vi "Main.vi"(8 "error in":errorcluster, 11 "Container in":refnum<class "Container.lvclass">) -> (0 "error out":errorcluster, 3 "Container out":refnum<class "Container.lvclass">)   [LabVIEW 2023, in "Container.lvclass"]
doc: "The Queued Message Handler of a Worker."
uses:
  Container.lvclass
  C:/Program Files (x86)/National Instruments/LabVIEW 2023/vi.lib/addons/_Workers/Library/Classes/Worker/Worker.lvclass
  System.Windows.Forms
  Container.lvclass/Container.ctl
  <vilib>/addons/_Workers/Library/Classes/Worker/Worker.lvclass/Worker.ctl
  Worker-1/Worker-1.lvclass
  <userlib>/LV-TOML/lib/Write TOML File (TOML).vi
  <vilib>/addons/_Workers/Library/Classes/Message/Enqueue Message to Queue.vi
  <vilib>/addons/_Workers/Library/Classes/Message/Enqueue Message to Self v2.vi
  <vilib>/MGI/Panel Manager - .NET Panels/MDI/MDI Container/MDI Container.lvclass
  <vilib>/MGI/Panel Manager/Panel/Panel/Window/Window.lvclass
  UI Cam Basler/UI Cam Basler.lvclass
  Initialization Data.ctl
  <vilib>/addons/_Workers/Library/Classes/Worker/Worker.lvclass
  <vilib>/addons/_Workers/Debugger/Debug Client/Debug Client.lvlib
  <vilib>/addons/_Workers/Library/Classes/Message/Message.lvclass
  <userlib>/LV-TOML/lib/LV-TOML.lvlib
  C:/Program Files (x86)/National Instruments/LabVIEW 2023/vi.lib/addons/_Workers/Library/Classes/Workers Object/Workers Object.lvclass
  C:/Users/flepetit/Desktop/CamView-mdi-LV/Workers/Container/Container.lvclass
  C:/Users/flepetit/Desktop/CamView-mdi-LV/Workers/Worker-1/Worker-1.lvclass
panel:
  in  "Camera monitoring container":refnum<k24>(container)
  out "Caméra CL":bool
  in  "Plac.Hor.":bool
  in  "Plac.Vert.":bool
  out "Caméra CP":bool
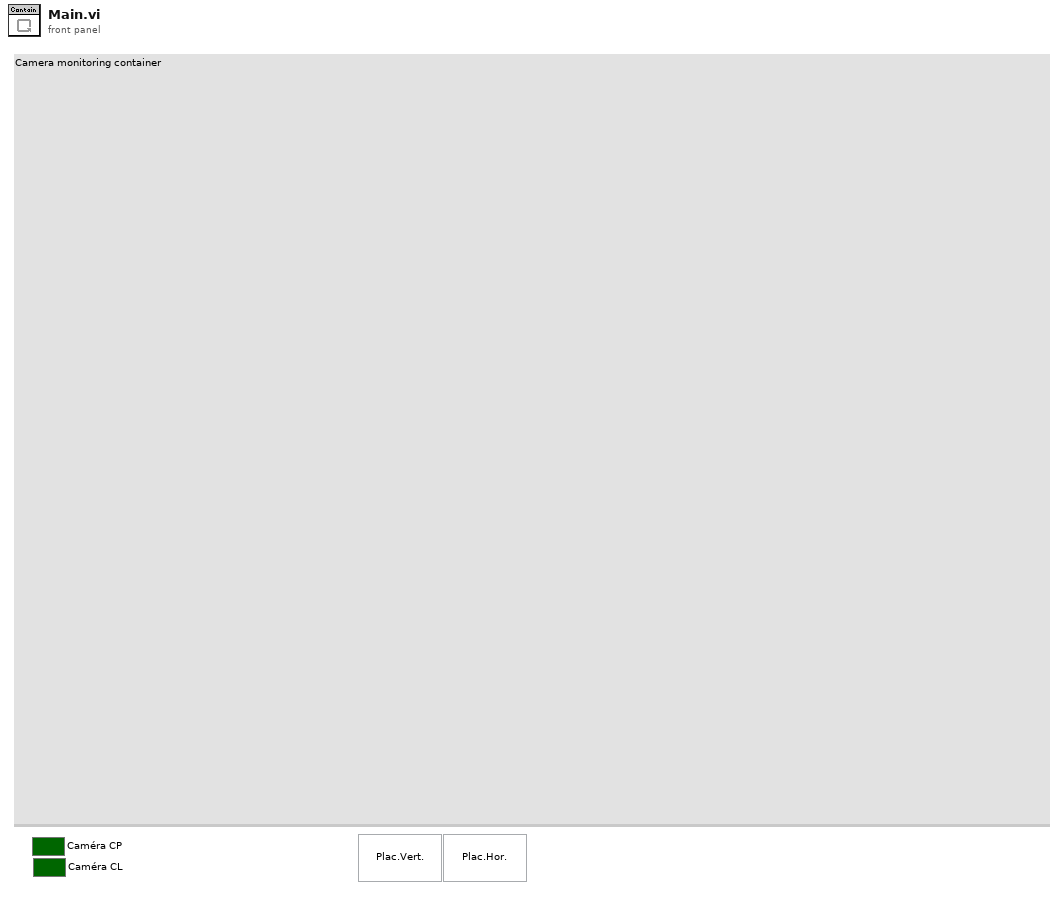
[diagram p1: front panel]
types:
  T1 = typedef "Container.lvclass/Initialization Data.ctl" = cluster{"String":string}
  T2 = typedef "Container.lvclass/Parsed data container.ctl" = cluster{"Ctrl Config":cluster{"Caméra CP":bool, "Caméra CL":bool}}
  T3 = typedef "LV-TOML.lvlib/TOML Value.ctl" = cluster{"type":enum16{"Table", "Array", "String", "Integer", "Float", "Boolean", "Offset Date-Time", "Local Date-Time", "Local Date", "Local Time", "Path"}, "value":variant}
  T4 = typedef "Workers.lvlib/Case Label.ctl" = string
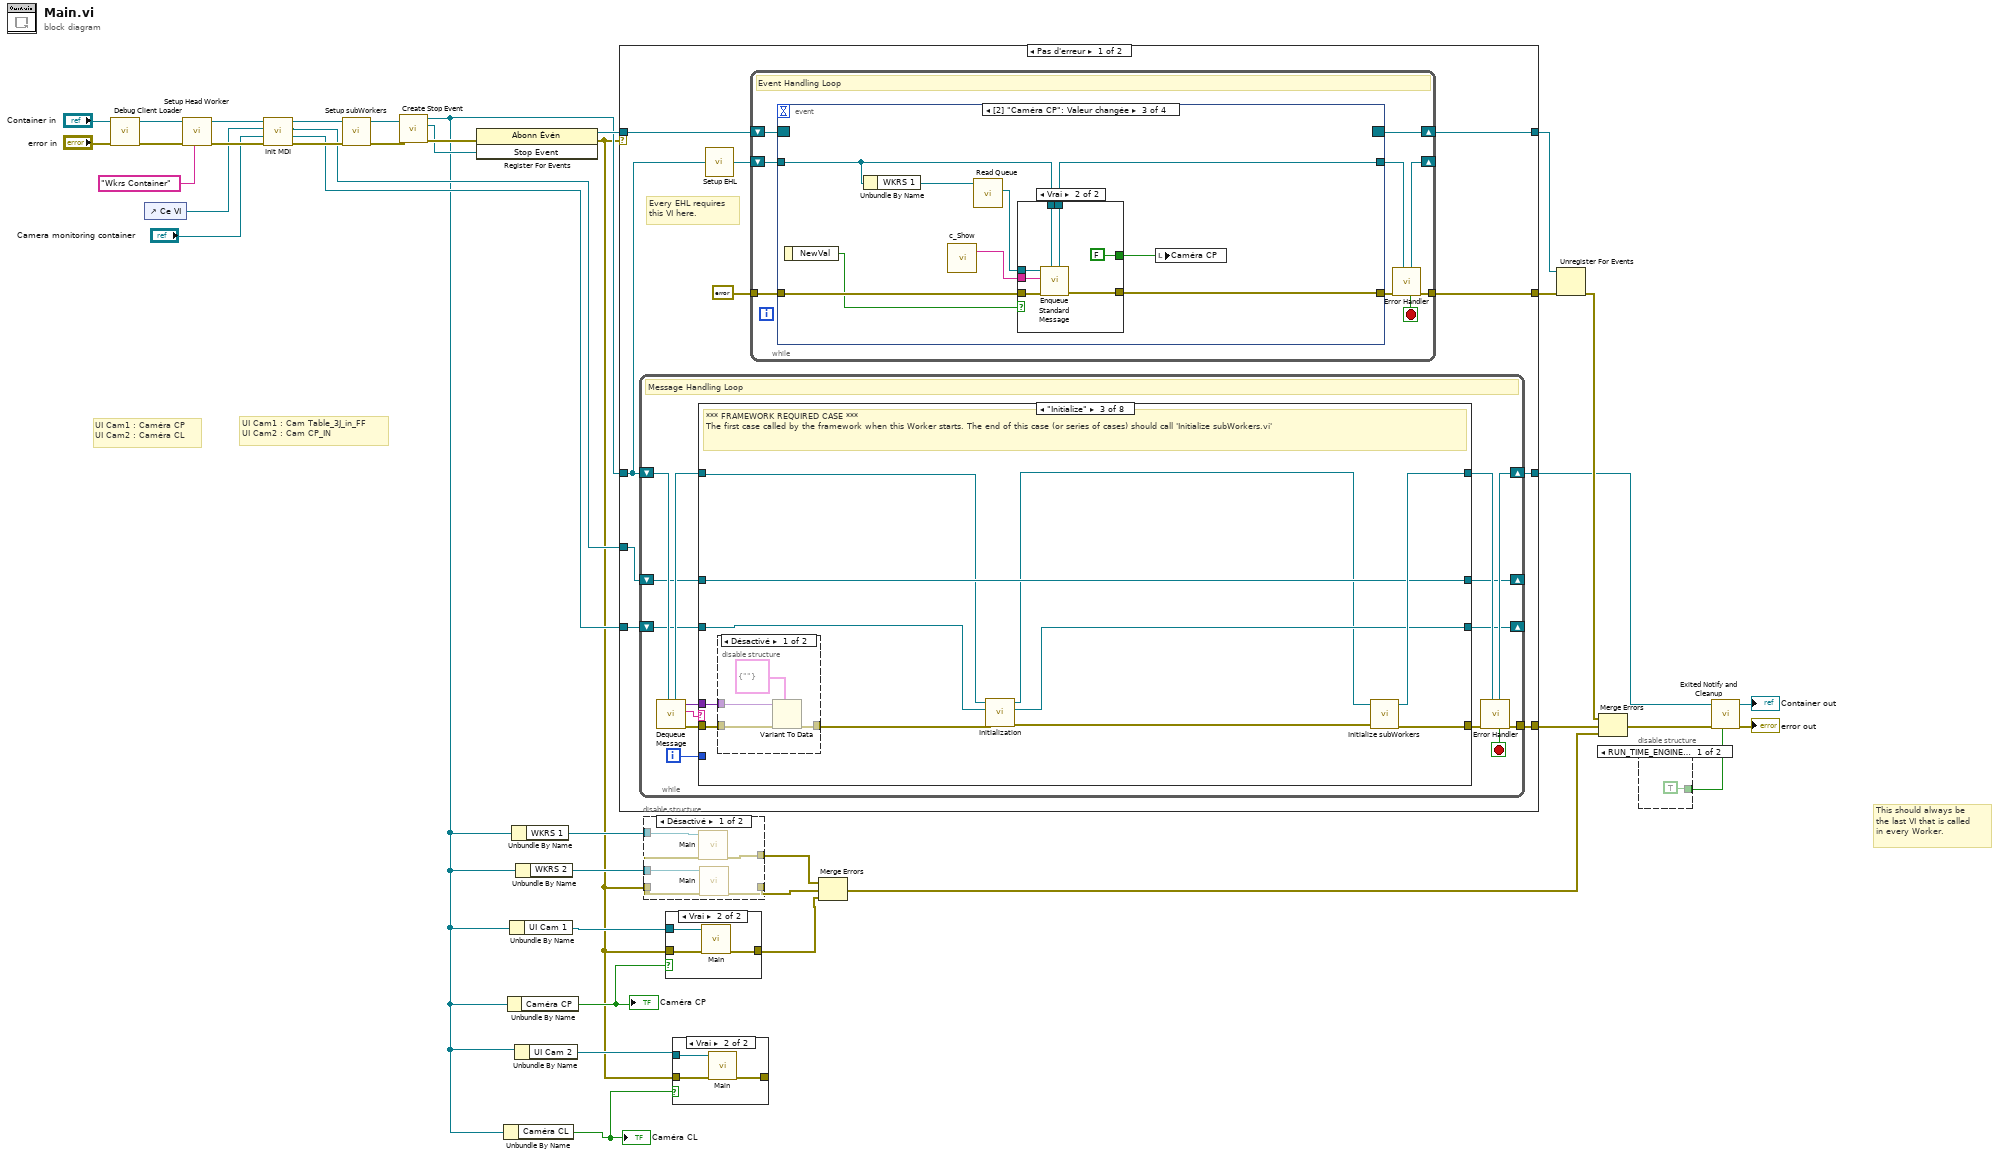
[diagram p0: block diagram]
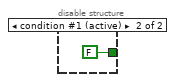
[diagram p2: hidden frame]
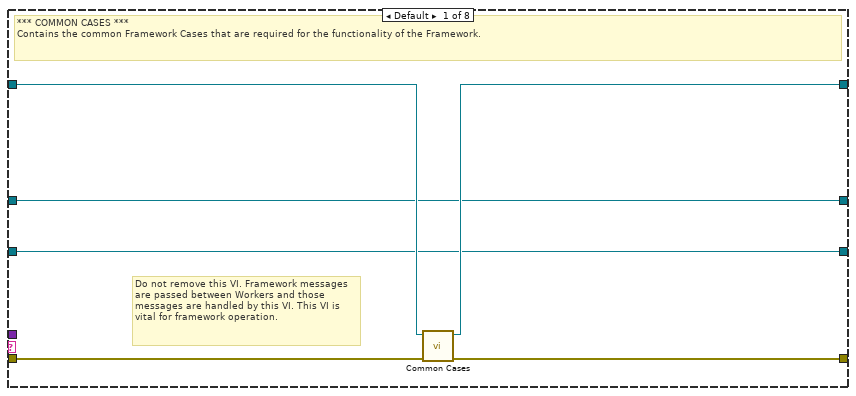
[diagram p6: hidden frame]
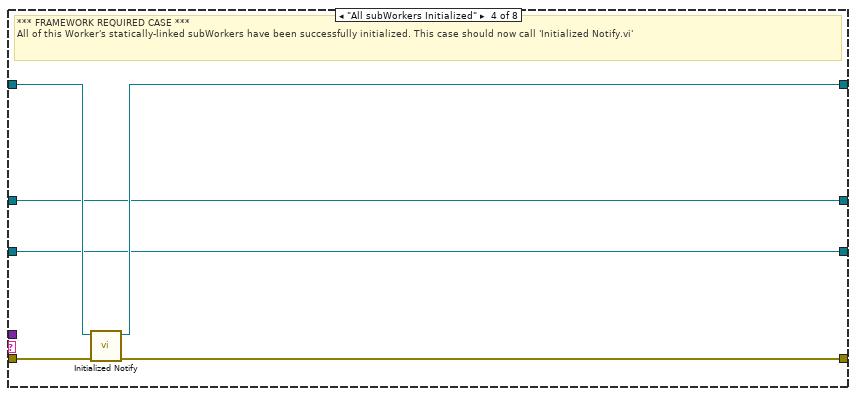
[diagram p9: hidden frame]
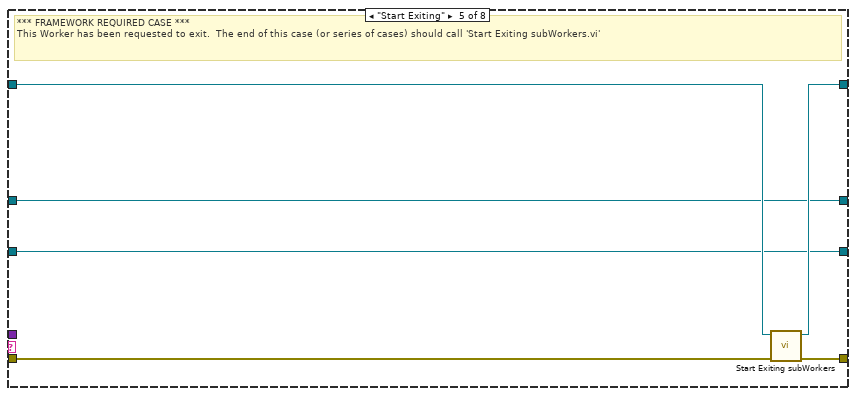
[diagram p10: hidden frame]
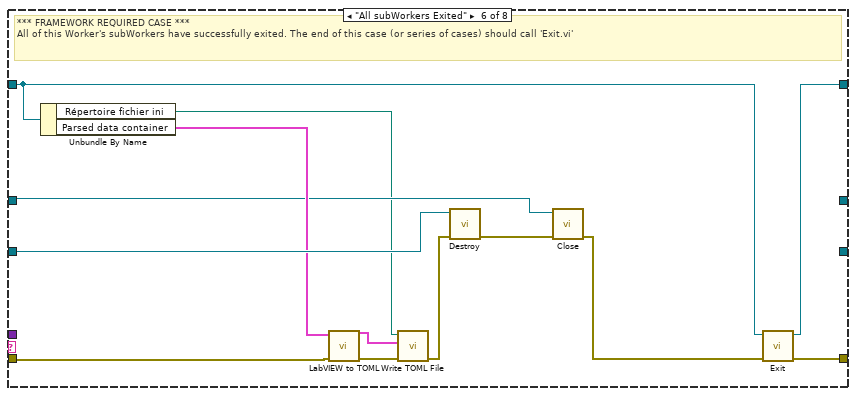
[diagram p11: hidden frame]
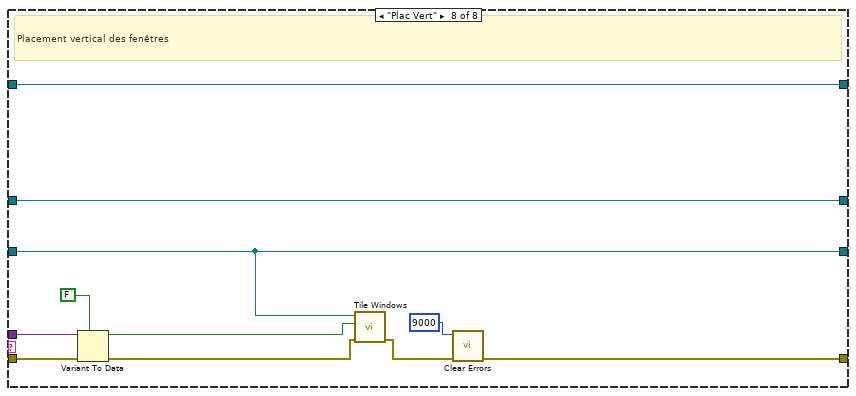
[diagram p13: hidden frame]
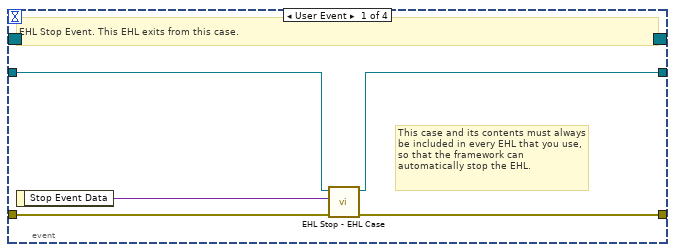
[diagram p14: hidden frame]
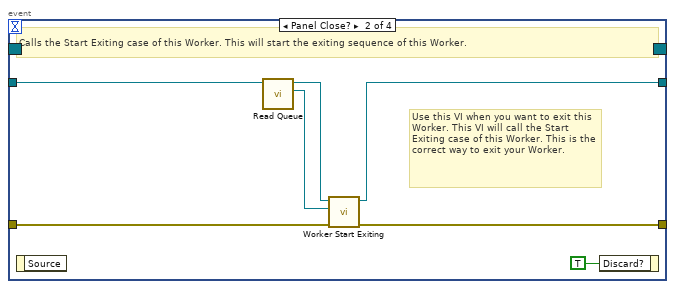
[diagram p15: hidden frame]
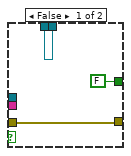
[diagram p16: hidden frame]
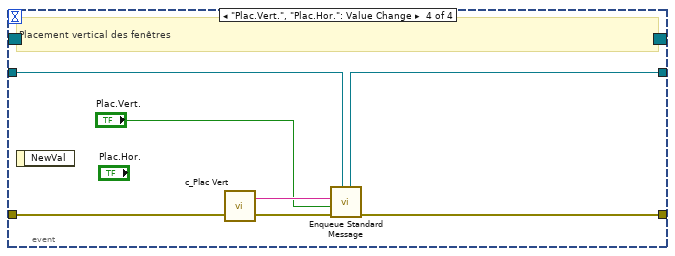
[diagram p17: hidden frame]
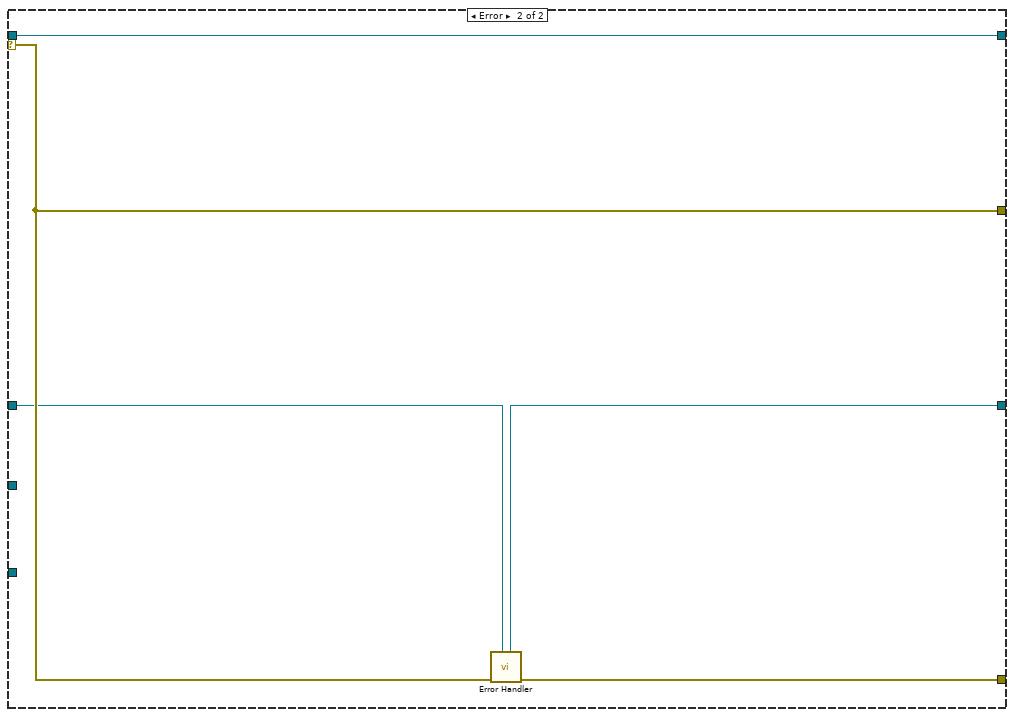
[diagram p18: hidden frame]
diagram:
  # "UI Cam1 : Cam Table_3J_in_FF\nUI Cam2 : Cam CP_IN"
  # "UI Cam1 : Caméra CP\nUI Cam2 : Caméra CL"
  # "This should always be the last VI that is called in every Worker."
  n1 = call <vilib>:"Debug Client Loader.vi"("error in (no error)"="error in", "Worker"="Container in") -> ("error out"=w24:errorcluster, "Worker out"=w23:refnum<class "Container.lvclass">)  [unwired: 8 in]
  n2 = control-ref of="Ce VI"() -> (w9:refnum<vi>)
  n3 = call-dynamic "Setup Head Worker.vi"("Worker Alias"="Wkrs Container", "error in"=w24, "Worker"=w23) -> ("error out"=w15:errorcluster, "Worker out"=w12:refnum<class "Container.lvclass">)  [unwired: 7 in]
  n4 = call "Init MDI.vi"("error in (no error)"=w15, "Camera monitoring container"="Camera monitoring container", "Refnum VI"=w9, "Container en entrée"=w12) -> ("error out"=w14:errorcluster, "Container out"=w10:refnum<class "MDI Container.lvclass">, "Panel Out"=w11:refnum<class "Window.lvclass">, "Container en sortie"=w13:refnum<class "Container.lvclass">)  [unwired: 4 in]
  n5 = call "Setup subWorkers.vi"("error in"=w14, "Container in"=w13) -> ("error out"=w21:errorcluster, "Container out"=w22:refnum<class "Container.lvclass">)  [unwired: 8 in]
  n6 = call-dynamic "Create Stop Event.vi"("error in"=w21, "Worker"=w22) -> ("error out"=w34:errorcluster, "Stop Event"=w31:refnum<user-event>, "Worker out"=w6:refnum<class "Container.lvclass">)  [unwired: 7 in]
  n7 = register-events(error in=w34, w31) -> (reference out=w33:refnum<event-registration>, error out=w4:errorcluster)  [unwired: 1 in]
  n8 = Unbundle By Name(w6) -> ("Caméra CL"=w3:bool)
  "Caméra CL" <- w3
  n9 = Unbundle By Name(w6) -> ("Caméra CP"=w7:bool)
  "Caméra CP" <- w7
  n10 = Unbundle By Name(w6) -> ("UI Cam 1"=w17:refnum<class "UI Cam Basler.lvclass">)
  n11 = Unbundle By Name(w6) -> ("WKRS 1"=w27:refnum<class "Worker-1.lvclass">)
  n12 = Unbundle By Name(w6) -> ("UI Cam 2"=w5:refnum<class "UI Cam Basler.lvclass">)
  n13 = Unbundle By Name(w6) -> ("WKRS 2"=w19:refnum<class "Worker-1.lvclass">)
  n14 = case shown="Pas d'erreur" w4 {
    tunnel: w6 -> [w44 w178]
    tunnel: [w42 w179] -> w32
    tunnel: w33 -> [w49 w180]
    tunnel: [w46 w181] -> w38
    tunnel: [w48 w180] -> w37
    tunnel: [w43 w177] -> w35
    selector: w4 -> [_ w181]
    tunnel: w11 -> [w41 _]
    tunnel: w10 -> [w40 _]
    frame No Error {
      # "Every EHL requires\nthis VI here."
      n15 = while {
        shift-right: [w62] -> w43
        shift-left: w44 -> [w64]
        tunnel: [w63] -> w42
        shift-right: [w53] -> _
        shift-left: w41 -> [w52]
        shift-right: [w51] -> _
        shift-left: w40 -> [w50]
        i -> [w54]
        stop <- w55 stop-if-true
        # "Message Handling Loop"
        n16 = call-dynamic "Dequeue Message.vi"("Worker"=w64) -> ("error out"=w61:errorcluster, "Case out"=w56:string, "Data out"=w57:variant, "Worker out"=w59:refnum<class "Container.lvclass">)  [unwired: 6 in, 1 out]
        n17 = case "Worker MHL Case Structure (DO NOT CHANGE LABEL NAME)" shown="\"Initialize\"" w56 {
          tunnel: w61 -> [w70 w73 w83 w94 w99 w108 w118 w128]
          tunnel: [w69 w73 w85 w93 w102 w115 w118 w121] -> w60
          tunnel: w59 -> [w68 w74 w76 w96 w100 w104 w119 w130]
          tunnel: [w67 w74 w84 w95 w101 w114 w119 w130] -> w58
          tunnel: w57 -> [_ _ w82 _ _ _ _ w127]
          tunnel: w54 -> [_ _ _ _ _ _ _ _]
          tunnel: [w66 w72 w81 w92 w98 _ w117 w129] -> w53
          tunnel: w52 -> [w66 w72 w81 w92 w98 w105 w117 w129]
          tunnel: [w65 w71 w77 w91 w97 _ w116 w120] -> w51
          tunnel: w50 -> [w65 w71 w78 w91 w97 w111 w116 w120]
          frame Default {
            # "Do not remove this VI. Framework messages are passed between Workers and those messages are handled by this VI. This VI is vital for framework operation."
            # "*** COMMON CASES ***\nContains the common Framework Cases that are required for the functionality of the Framework."
            n18 = call-dynamic "Common Cases.vi"("error in"=w70, "Worker in"=w68) -> ("error out"=w69:errorcluster, "Worker out"=w67:refnum<class "Container.lvclass">)  [unwired: 8 in]
          }
          frame "------ FRAMEWORK REQUIRED CASES ------" {
            # "Start of Framework Required Cases"
          }
          frame "Initialize" {
            # "*** FRAMEWORK REQUIRED CASE ***\nThe first case called by the framework when this Worker starts. The end of this case (or series of cases) should call 'Initialize subWorkers.vi'"
            n19 = disable-structure shown="Désactivé" {
              disable-tunnel: w83 -> [w89 w90]
              disable-tunnel: [w88 w90] -> w80
              disable-tunnel: w82 -> [w87 _]
              frame Disabled {
                n20 = Variant To Data(error in=w89, type=T1 {"String"=""} ("Initialization Data"), Variant=w87) -> (error out=w88:errorcluster)  [unwired: 1 out]
              }
              frame Enabled {
              }
            }
            n21 = call "Initialization.vi"("error in (no error)"=w80, "Container in"=w78, "Container en entrée"=w76) -> ("error out"=w79:errorcluster, "Container out"=w77:refnum<class "MDI Container.lvclass">, "Container en sortie"=w75:refnum<class "Container.lvclass">)  [unwired: 6 in]
            n22 = call-dynamic "Initialize subWorkers.vi"("error in"=w79, "Worker"=w75) -> ("error out"=w85:errorcluster, "dup Worker out"=w84:refnum<class "Container.lvclass">)  [unwired: 8 in]
          }
          frame "All subWorkers Initialized" {
            # "*** FRAMEWORK REQUIRED CASE ***\nAll of this Worker's statically-linked subWorkers have been successfully initialized. This case should now call 'Initialized Notify.vi'"
            n23 = call-dynamic "Initialized Notify.vi"("error in"=w94, "Worker"=w96) -> ("error out"=w93:errorcluster, "dup Worker out"=w95:refnum<class "Container.lvclass">)  [unwired: 8 in]
          }
          frame "Start Exiting" {
            # "*** FRAMEWORK REQUIRED CASE ***\nThis Worker has been requested to exit.  The end of this case (or series of cases) should call 'Start Exiting subWorkers.vi'"
            n24 = call-dynamic "Start Exiting subWorkers.vi"("error_in"=w99, "Worker"=w100) -> ("error out"=w102:errorcluster, "dup Worker out"=w101:refnum<class "Container.lvclass">)  [unwired: 8 in]
          }
          frame "All subWorkers Exited" {
            # "*** FRAMEWORK REQUIRED CASE ***\nAll of this Worker's subWorkers have successfully exited. The end of this case (or series of cases) should call 'Exit.vi'"
            n25 = Unbundle By Name(w104) -> ("Répertoire fichier ini"=w103:path, "Parsed data container"=w106:T2)
            n26 = call <userlib>:"LabVIEW to TOML.vi"("error in (no error)"=w108, "LV Value"=w106) -> ("error out"=w109:errorcluster, "TOML Value"=w110:T3)  [unwired: 7 in, 1 out]
            n27 = call-poly <userlib>:"Write TOML File.vi"("error in (no error)"=w109, "Value"=w110, "file path (use dialog)"=w103) -> ("error out"=w107:errorcluster)  [unwired: 8 in]
            n28 = call <vilib>:"Destroy.vi"("error in (no error)"=w107, "Container in"=w111) -> ("error out"=w113:errorcluster)  [unwired: 9 in]
            n29 = call-dynamic "Close.vi"("error in (no error)"=w113, "UI Element in"=w105) -> ("error out"=w112:errorcluster)  [unwired: 9 in]
            n30 = call-dynamic "Exit.vi"("error_in"=w112, "Worker"=w104) -> ("error out"=w115:errorcluster, "dup Worker out"=w114:refnum<class "Container.lvclass">)  [unwired: 8 in]
          }
          frame "------------------Himself---------------------------" {
            # "End of Framework Required Cases"
          }
          frame "Plac Vert" {
            # "Placement vertical des fenêtres"
            n31 = Variant To Data(error in=w128, type=FALSE, Variant=w127) -> (data=w125:bool, error out=w124:errorcluster)
            n32 = call <vilib>:"Tile Windows.vi"("error in (no error)"=w124, "Vertical?"=w125, "Container in"=w120) -> ("error out"=w122:errorcluster)  [unwired: 8 in]
            n33 = call <vilib>:"Clear Errors.vi"("error in (no error)"=w122, "specific error code to clear (0: all)"=9000) -> ("error out"=w121:errorcluster)  [unwired: 4 in, 1 out]
          }
        }
        n34 = call-dynamic "Error Handler.vi"("Worker"=w58, "error_in"=w60) -> ("error out"=w63:errorcluster, "Stop Loop"=w55:bool, "Worker out"=w62:refnum<class "Container.lvclass">)  [unwired: 7 in]
      }
      n35 = call-dynamic "Setup EHL.vi"("Worker"=w44) -> ("Worker out"=w45:refnum<class "Container.lvclass">)  [unwired: 14 in]
      n36 = while "Event Handling Loop" {
        shift-right: [w139] -> w48
        shift-left: w49 -> [w138]
        tunnel: [w134] -> w46
        tunnel: errorcluster {"status"=FALSE, "code"=0, "source"=""} ("error constant") -> [w136]
        shift-right: [w132] -> _
        shift-left: w45 -> [w137]
        stop <- w131 stop-if-true
        # "Event Handling Loop"
        n37 = event shown="[2] \"Caméra CP\": Valeur changée" {
          selector: w138 -> [_ _ _ _]
          dyn-events: [_ _ _ _] -> w139
          timeout: _ -> [_ _ _ _]
          tunnel: [w143 w150 w158 w173] -> w135
          tunnel: w136 -> [w144 w149 w160 w174]
          tunnel: w137 -> [w142 w148 w157 w176]
          tunnel: [w141 w147 w159 w175] -> w133
          event User Event {
            # "This case and its contents must always be included in every EHL that you use, so that the framework can automatically stop the EHL."
            # "EHL Stop Event. This EHL exits from this case."
            n38 = event-data() -> ("Stop Event Data"=w140:variant)  [unwired: 1 in]
            n39 = call <vilib>:"EHL Stop - EHL Case.vi"("error in"=w144, "Stop Event Data"=w140, "Worker"=w142) -> ("error out"=w143:errorcluster, "Worker out"=w141:refnum<class "Container.lvclass">)  [unwired: 7 in]
          }
          event Panel Close? {
            # "Use this VI when you want to exit this Worker. This VI will call the Start Exiting case of this Worker. This is the correct way to exit your Worker."
            # "Calls the Start Exiting case of this Worker. This will start the exiting sequence of this Worker."
            n40 = event-data() -> ()  [unwired: 1 in, 1 out]
            n41 = call <vilib>:"Read Queue.vi"("Worker"=w148) -> ("Message Queue out"=w145:refnum<class "Message Queue.lvclass">, "dup Worker out"=w146:refnum<class "Container.lvclass">)  [unwired: 9 in]
            n42 = call-dynamic "Worker Start Exiting.vi"("error_in"=w149, "Message Queue"=w145, "Worker"=w146) -> ("error out"=w150:errorcluster, "dup Worker out"=w147:refnum<class "Container.lvclass">)  [unwired: 7 in]
            n43 = event-data ("Nœud de filtre d'événements")("Discard?"=TRUE) -> ()  [unwired: 1 in, 1 out]
          }
          event "Caméra CP": Value Change {
            n44 = event-data() -> ("NewVal"=w153:bool)  [unwired: 1 in]
            n45 = Unbundle By Name(w157) -> ("WKRS 1"=w156:refnum<class "Worker-1.lvclass">)
            n46 = call "c_Show.vi"() -> ("Case Label"=w154:T4)  [unwired: 1 in]
            n47 = call <vilib>:"Read Queue.vi"("Worker"=w156) -> ("Message Queue out"=w155:refnum<class "Message Queue.lvclass">)  [unwired: 9 in, 1 out]
            n48 = case shown="Vrai" w153 {
              tunnel: w160 -> [w163 w170]
              tunnel: [w162 w169] -> w159
              tunnel: [w163 w168] -> w158
              tunnel: w157 -> [w162 w167]
              tunnel: w155 -> [_ w166]
              tunnel: w154 -> [_ w165]
              tunnel: [FALSE FALSE] -> w152
              frame False {
              }
              frame True {
                n49 = call-poly <vilib>:"Enqueue Standard Message.vi"("Worker"=w167, "error in"=w170, "Case Label"=w165, "Message Queue"=w166) -> ("error out"=w168:errorcluster, "dup Worker out"=w169:refnum<class "Container.lvclass">)  [unwired: 5 in, 1 out]
              }
            }
            n50 = local write "Caméra CP"(w152) -> ()
          }
          event "Plac.Vert.", "Plac.Hor.": Value Change {
            # "Placement vertical des fenêtres"
            n51 = event-data() -> ()  [unwired: 1 in, 1 out]
            n52 = call "c_Plac Vert.vi"() -> ("Case Label"=w172:T4)  [unwired: 1 in]
            n53 = call-poly <vilib>:"Enqueue Standard Message.vi"("Worker"=w176, "error in"=w174, "Data"="Plac.Vert.", "Case Label"=w172) -> ("error out"=w173:errorcluster, "dup Worker out"=w175:refnum<class "Container.lvclass">)  [unwired: 6 in]
          }
        }
        n54 = call-dynamic "Error Handler.vi"("Worker"=w133, "error_in"=w135) -> ("error out"=w134:errorcluster, "Stop Loop"=w131:bool, "Worker out"=w132:refnum<class "Container.lvclass">)  [unwired: 7 in]
      }
    }
    frame Error {
      n55 = call-dynamic "Error Handler.vi"("Worker"=w178, "error_in"=w181) -> ("error out"=w179:errorcluster, "Worker out"=w177:refnum<class "Container.lvclass">)  [unwired: 7 in, 1 out]
    }
  }
  n56 = disable-structure shown="Désactivé" {
    disable-tunnel: [w186 _] -> w29
    disable-tunnel: w27 -> [w185 _]
    disable-tunnel: w19 -> [w184 _]
    disable-tunnel: [w183 _] -> w18
    disable-tunnel: w4 -> [w182 _]
    frame Disabled {
      n57 = call-dynamic "Main.vi"("error in"=w182, "Worker-1 in"=w185) -> ("error out"=w186:errorcluster)  [unwired: 8 in, 1 out]
      n58 = call-dynamic "Main.vi"("error in"=w182, "Worker-1 in"=w184) -> ("error out"=w183:errorcluster)  [unwired: 8 in, 1 out]
    }
    frame Enabled {
    }
  }
  n59 = case shown="Vrai" w7 {
    tunnel: w17 -> [_ w190]
    tunnel: w4 -> [w187 w189]
    tunnel: [w187 w188] -> w16
    frame False {
    }
    frame True {
      n60 = call-dynamic "Main.vi"("error in"=w189, "UI Cam Basler in"=w190) -> ("error out"=w188:errorcluster)  [unwired: 8 in, 1 out]
    }
  }
  n61 = case shown="Vrai" w3 {
    tunnel: w5 -> [_ w194]
    tunnel: w4 -> [w191 w193]
    tunnel: [w191 w192] -> _
    frame False {
    }
    frame True {
      n62 = call-dynamic "Main.vi"("error in"=w193, "UI Cam Basler in"=w194) -> ("error out"=w192:errorcluster)  [unwired: 8 in, 1 out]
    }
  }
  n63 = Merge Errors(w29, w18, w16) -> (w28:errorcluster)
  n64 = Unregister For Events(event registration refnum=w37, error in=w38) -> (error out=w39:errorcluster)
  n65 = Merge Errors ("Fusionner les erreurs")(w39, w32, w28) -> (w36:errorcluster)
  n66 = disable-structure shown="RUN_TIME_ENGINE==True" {
    disable-tunnel: [TRUE ("Close FP on Exit? (T)") FALSE ("Close FP on Exit? (T)")] -> w2
    frame condition #0 {
    }
    frame condition #1 (active) {
    }
  }
  n67 = call-dynamic "Exited Notify and Cleanup.vi"("Close FP on Exit? (T)"=w2, "error_in"=w36, "Worker"=w35) -> ("error out"=→"error out":errorcluster, "dup Worker out"=→"Container out":refnum<class "Container.lvclass">)  [unwired: 7 in]
